vi "Parse API GET Filter Parameters.vi"(8 "error in (no error)":errorcluster, 9 "Parameters Names":T2, 10 "Parameters Collection Name":string="formInput", 11 "Response Body in":string) -> (0 "error out":errorcluster, 2 "Parameters Values":T1, 3 "Response Body out":string)   [LabVIEW 2017]
uses:
  Types/Parameters Names Type.ctl
  Types/Parameters Values Type.ctl
  <vilib>/LVH/i3 JSON/JSON Parsing/Get Object Parameter Files/Get Object Parameter - Object.vi
  <vilib>/LVH/i3 JSON/i3-json.lvlib
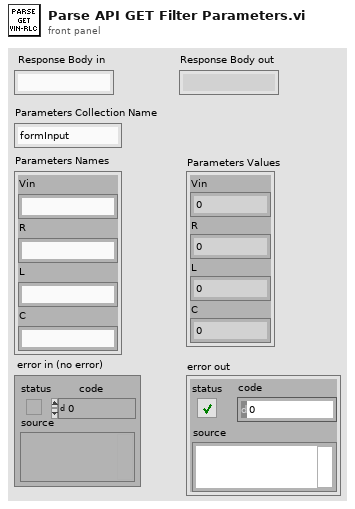
[diagram p1: front panel]
types:
  T1 = typedef "Parameters Values Type.ctl" = cluster{"Vin":dbl, "R":dbl, "L":dbl, "C":dbl}
  T2 = typedef "Parameters Names Type.ctl" = cluster{"Vin":string, "R":string, "L":string, "C":string}
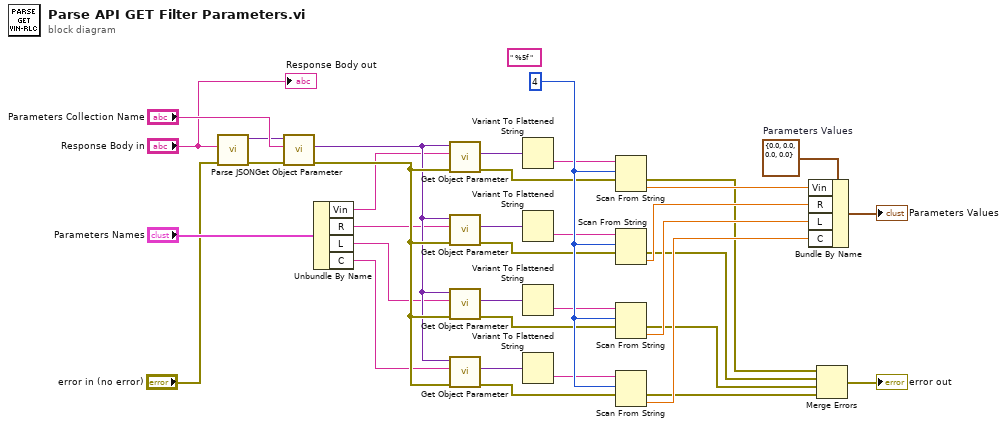
[diagram p0: block diagram]
diagram:
  w15 = T1 {"Vin"=0.0, "R"=0.0, "L"=0.0, "C"=0.0}  # Parameters Values
  w22 = u32 4 ("initial scan location")
  (unwired) " %5f " ("format string")
  n1 = call <vilib>:"Parse JSON.vi"("error in (no error)"="error in (no error)", "JSON String"="Response Body in") -> ("error out"=w33:errorcluster, "JSON Tree"=w35:variant)  [unwired: 6 in, 2 out]
  n2 = call-poly <vilib>:"Get Object Parameter.vi"("error in (no error)"=w33, "Parameter Name"="Parameters Collection Name", "JSON Tree In (JSON Object)"=w35) -> ("error out"=w32:errorcluster, "JSON Object"=w31:variant)  [unwired: 5 in, 2 out]
  n3 = Unbundle By Name("Parameters Names") -> ("Vin"=w30:string, "R"=w29:string, "L"=w28:string, "C"=w27:string)
  n4 = call-poly <vilib>:"Get Object Parameter.vi"("error in (no error)"=w32, "Parameter Name"=w30, "JSON Tree In (JSON Object)"=w31) -> ("error out"=w17:errorcluster, "JSON Object"=w23:variant)  [unwired: 5 in, 2 out]
  n5 = call-poly <vilib>:"Get Object Parameter.vi"("error in (no error)"=w32, "Parameter Name"=w29, "JSON Tree In (JSON Object)"=w31) -> ("error out"=w10:errorcluster, "JSON Object"=w24:variant)  [unwired: 5 in, 2 out]
  n6 = call-poly <vilib>:"Get Object Parameter.vi"("error in (no error)"=w32, "Parameter Name"=w28, "JSON Tree In (JSON Object)"=w31) -> ("error out"=w9:errorcluster, "JSON Object"=w25:variant)  [unwired: 5 in, 2 out]
  n7 = call-poly <vilib>:"Get Object Parameter.vi"("error in (no error)"=w32, "Parameter Name"=w27, "JSON Tree In (JSON Object)"=w31) -> ("error out"=w8:errorcluster, "JSON Object"=w26:variant)  [unwired: 5 in, 2 out]
  n8 = Variant To Flattened String(Variant=w23) -> (data string=w21:string)  [unwired: 1 out]
  n9 = Variant To Flattened String(Variant=w24) -> (data string=w20:string)  [unwired: 1 out]
  n10 = Variant To Flattened String(Variant=w25) -> (data string=w19:string)  [unwired: 1 out]
  n11 = Variant To Flattened String(Variant=w26) -> (data string=w18:string)  [unwired: 1 out]
  n12 = Scan From String(input string=w21, initial scan location=w22, error in=w17) -> (error out=w7:errorcluster, output 1=w14:dbl)  [unwired: 2 in, 2 out]
  n13 = Scan From String(input string=w20, initial scan location=w22, error in=w10) -> (error out=w6:errorcluster, output 1=w13:dbl)  [unwired: 2 in, 2 out]
  n14 = Scan From String(input string=w19, initial scan location=w22, error in=w9) -> (error out=w5:errorcluster, output 1=w12:dbl)  [unwired: 2 in, 2 out]
  n15 = Scan From String(input string=w18, initial scan location=w22, error in=w8) -> (error out=w4:errorcluster, output 1=w11:dbl)  [unwired: 2 in, 2 out]
  n16 = Bundle By Name(cluster=w15, "Vin"=w14, "R"=w13, "L"=w12, "C"=w11) -> (→"Parameters Values":T1)
  n17 = Merge Errors(w7, w6, w5, w4) -> (→"error out":errorcluster)
  "Response Body out" <- "Response Body in"
